vi "Ctor.vi"(8 "error in (no error)":errorcluster, 10 "Starting Users (None)":refnum<class "User.lvclass">[](array[class])) -> (0 "error out":errorcluster, 3 "InMemoryUserProvider out":refnum<class "InMemoryUserProvider.lvclass">)   [LabVIEW 2020, in "HTTP Server.lvlib" / "InMemoryUserProvider.lvclass"]
uses:
  InMemoryUserProvider.lvclass
  User/User.lvclass
  InMemoryUserProvider.lvclass/InMemoryUserProvider.ctl
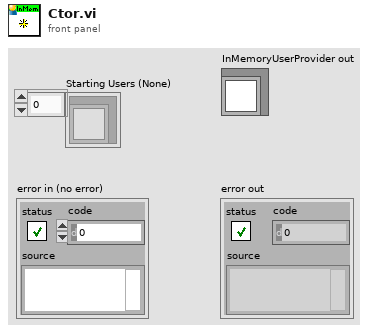
[diagram p1: front panel]
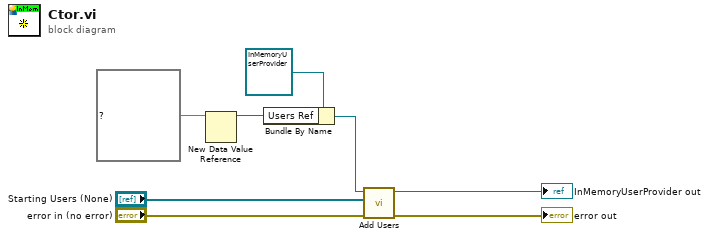
[diagram p0: block diagram]
diagram:
  n1 = New Data Value Reference(data value=map{string, refnum<class "User.lvclass">} {} ("Users")) -> (data value reference=w6:refnum<data-value>)  [unwired: 1 in, 1 out]
  n2 = Bundle By Name(cluster=refnum<class "InMemoryUserProvider.lvclass"> refnum ("InMemoryUserProvider in"), "Users Ref"=w6) -> (w5:refnum<class "InMemoryUserProvider.lvclass">)
  n3 = call "Add Users.vi"("error in (no error)"="error in (no error)", "Users"="Starting Users (None)", "InMemoryUserProvider in"=w5) -> ("error out"=→"error out":errorcluster, "InMemoryUserProvider out"=→"InMemoryUserProvider out":refnum<class "InMemoryUserProvider.lvclass">)  [unwired: 7 in]
